vi "DataEntryTransform.vi"(7 "DataTrasform":T5, 8 "Error In":errorcluster, 9 "AnalysisStepName":string, 10 "MainSettingIn":T3, 11 "CoordSettingIn":T1 {"ROI"."Contours"."Type" items=["No Selection", "Point", "Line", "Rectangle", "Oval", "Polygon", "Freehand Region", "Annulus", "Unused2", "Unused3", "Broken Line", "Freehand Line", "Rotated Rectangle"]}) -> (0 "Error Out":errorcluster, 2 "CoordSettingOut":T1 {"ROI"."Contours"."Type" items=["No Selection", "Point", "Line", "Rectangle", "Oval", "Polygon", "Freehand Region", "Annulus", "Unused2", "Unused3", "Broken Line", "Freehand Line", "Rotated Rectangle"]}, 3 "MainSettingOut":T3)   [LabVIEW 2019]
uses:
  Analysis/Controls/Analysis_Type.ctl
  Analysis/Controls/Analysis_Setting.ctl
  Control/DataTransform.ctl
  Control/CoordinateAnalysisSetting.ctl
  Analysis/Controls/V_Analysis_Type.ctl
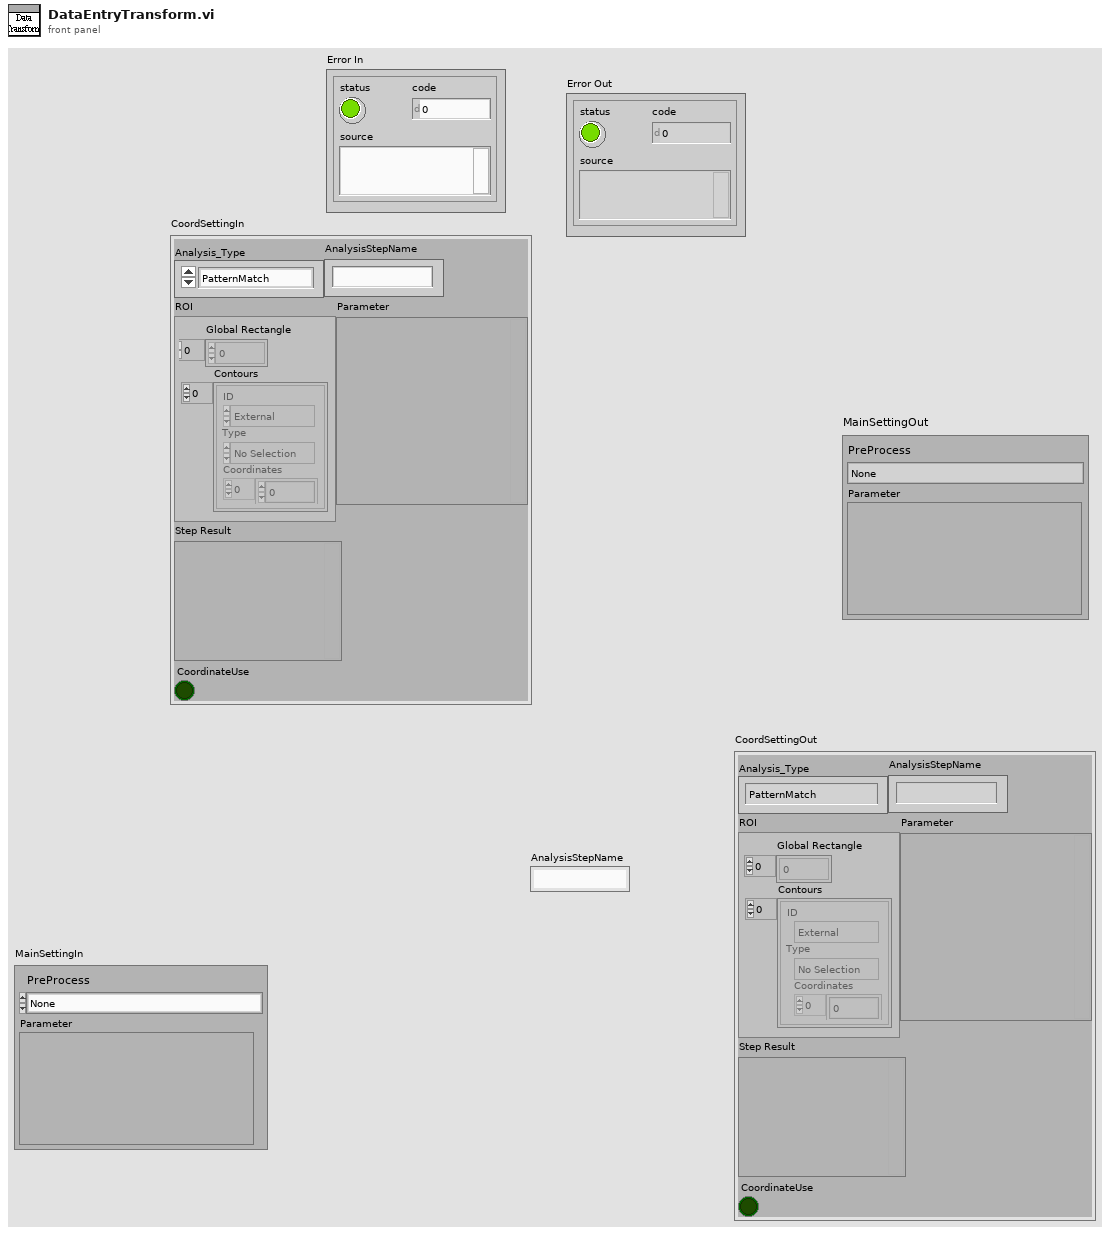
[diagram p1: front panel]
types:
  T1 = typedef "CoordinateAnalysisSetting.ctl" = cluster{"Analysis_Type":enum16{"PatternMatch", "Straight Edge"}, "ROI ":T2, "Parameter":variant, "Step Result":variant, "AnalysisStepName":string, "CoordinateUse":bool}
  T2 = typedef "ROI Descriptor" = cluster{"Global Rectangle":i32[], "Contours":cluster{"ID":enum32{"External", "Internal"}, "Type":u32, "Coordinates":i32[]}[]}
  T3 = typedef "Analysis_Setting.ctl" = cluster{"PreProcess":T4, "Parameter":string}
  T4 = typedef "V_Analysis_Type.ctl" = enum16{"None", "C_Color Pattern Matching", "G_PatternMatching", "G_ShapeDectect"}
  T5 = typedef "DataTransform.ctl" = enum16{"CoordToMain", "MainToCoord"}
  T6 = typedef "Analysis_Type.ctl" = u16
  T7 = cluster{"ID":enum32{"External", "Internal"}, "Type":u32, "Coordinates":i32[]}[]
  T8 = cluster{"ID":enum32{"External", "Internal"}, "Type":u32, "Coordinates":i32[]}
  T9 = cluster{"Analysis_Type":T6, cluster{"ID":enum32{"External", "Internal"}, "Type":u32, "Coordinates":i32[]}, "Parameter":variant}
  T10 = cluster{"Contour Type":u32, "ROI Type":u32, "Points":i32[]}
  T11 = cluster{"Contour Type":u32, "ROI Type":u32, "Points":i32[]}[]
  T12 = cluster{"Points":i32[], cluster{"Contour Type":u32, "ROI Type":u32, "Points":i32[]}[]}
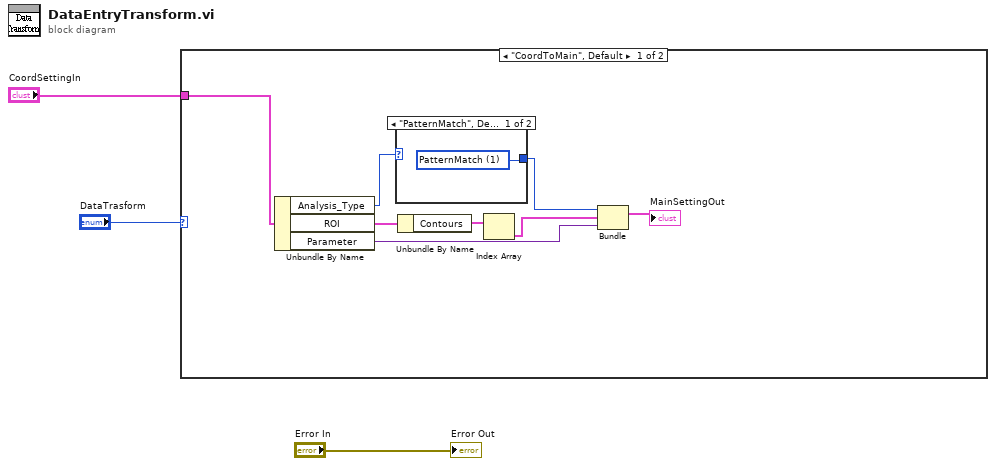
[diagram p0: block diagram]
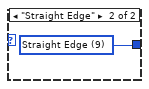
[diagram p2: hidden frame]
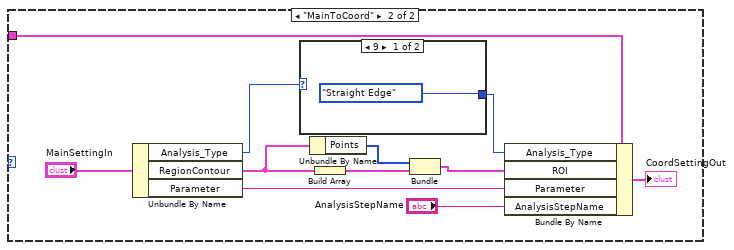
[diagram p3: hidden frame]
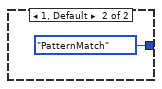
[diagram p4: hidden frame]
diagram:
  n1 = case shown="\"CoordToMain\", Default" "DataTrasform" {
    tunnel: "CoordSettingIn" -> [w4 w19]
    frame "CoordToMain", Default {
      n2 = Unbundle By Name(w4) -> ("Analysis_Type"=w7:enum16{"PatternMatch", "Straight Edge"}, "ROI"=w11:T2, "Parameter"=w8:variant)
      n3 = case shown="\"PatternMatch\", Default" w7 {
        tunnel: [w12 w13] -> w6
        frame "PatternMatch", Default {
          w12 = T6 1 items=["None", "PatternMatch", "Edge Detection", "Barcode 1D", "Barcode 2D", "Clamp", "Clamp MAX", "Particle", "Histogram", "Straight Edge", "Circle", "Shape Dectect", "OCR"] ("Analysis_Type")
        }
        frame "Straight Edge" {
          w13 = T6 9 items=["None", "PatternMatch", "Edge Detection", "Barcode 1D", "Barcode 2D", "Clamp", "Clamp MAX", "Particle", "Histogram", "Straight Edge", "Circle", "Shape Dectect", "OCR"] ("Analysis_Type")
        }
      }
      n4 = Unbundle By Name(w11) -> ("Contours"=w10:T7)
      n5 = Index Array(array=w10) -> (element=w9:T8)  [unwired: 1 in]
      n6 = Bundle("Analysis_Type"=w6, w9, "Parameter"=w8) -> (→"MainSettingOut":T9)  [unwired: 1 in]
    }
    frame "MainToCoord" {
      n7 = Unbundle By Name("MainSettingIn") -> ("Analysis_Type"=w23:T6, "RegionContour"=w21:T10, "Parameter"=w17:string)
      n8 = case shown="9" w23 {
        tunnel: [enum16{"PatternMatch", "Straight Edge"}."Straight Edge" ("Analysis_Type") enum16{"PatternMatch", "Straight Edge"}."PatternMatch" ("Analysis_Type")] -> w14
        frame 9 {
        }
        frame 1, Default {
        }
      }
      n9 = Unbundle By Name(w21) -> ("Points"=w22:i32[])
      n10 = Build Array(w21) -> (w20:T11)
      n11 = Bundle("Points"=w22, w20) -> (w18:T12)  [unwired: 1 in]
      n12 = Bundle By Name(cluster=w19, "Analysis_Type"=w14, "ROI"=w18, "Parameter"=w17, "AnalysisStepName"="AnalysisStepName") -> (→"CoordSettingOut":T1)
    }
  }
  "Error Out" <- "Error In"
